vi "Initialize Plot.vi"(8 "error in (no error)":errorcluster, 10 "scale (1)":dbl=1.0, 11 "serial arm in":refnum<class "NI_Robotics_Serial Robot Arm.lvclass">) -> (0 "error out":errorcluster, 3 "serial arm out":refnum<class "NI_Robotics_Serial Robot Arm.lvclass">)   [LabVIEW 2017, in "NI_Robotics_3DKinematics.lvlib"]
doc: "Initializes a 3D object that represents a robotic arm."
uses:
  <vilib>/robotics/Kinematics/Plotting/NI_Robotics_3DKinematics.lvlib
  <vilib>/robotics/Kinematics/Robot/NI_Robotics_Serial Robot Arm.lvclass
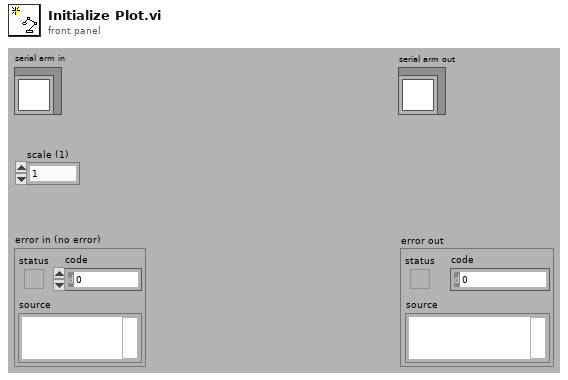
[diagram p1: front panel]
types:
  T1 = typedef "NI_Robotics_3DKinematics.lvlib/Tree Element.ctl" = cluster{"Name":string, "Parent":string, "Type":T2, "Visible?":bool, "Geometry Definition":dbl[], "Position WRT Parent (X,Y,Z)":dbl[], "Rotation WRT Parent (degrees)":dbl[], "Joint Type":T3, "Geometry File Path":path, "Indent Level":i32, "Color":u32}
  T2 = typedef "NI_Robotics_3DKinematics.lvlib/Element Type.ctl" = enum16{"Joint", "Box", "Cylinder", "Cone", "Sphere", "ASE File", "VRML File", "STL File", "Space"}
  T3 = typedef "NI_Robotics_3DKinematics.lvlib/Joint Type.ctl" = enum16{"Trans_X", "Trans_Y", "Trans_Z", "Rot_X", "Rot_Y", "Rot_Z", "None"}
  T4 = typedef "NI_Robotics_3DKinematics.lvlib/Joint Control.ctl" = cluster{"Joint Refnum":refnum<vi>, "Joint Type":T3, "Position WRT Parent":dbl[], "Rotation WRT Parent":dbl[], "Bar Refnum":refnum<vi>}
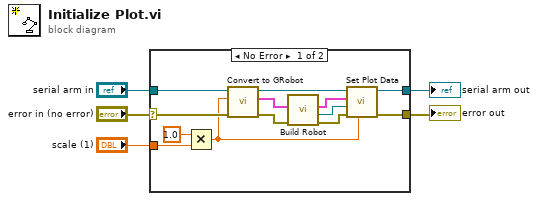
[diagram p0: block diagram]
diagram:
  n1 = case shown="No Error" "error in (no error)" {
    selector: "error in (no error)" -> [w13 w19]
    tunnel: "serial arm in" -> [w16 w20]
    tunnel: "scale (1)" -> [w14 _]
    tunnel: [w11 w19] -> w2
    tunnel: [w8 w20] -> w1
    frame No Error {
      n2 = Multiply(x=1.0, y=w14) -> (x*y=w6:dbl)
      n3 = call <vilib>:"Convert to GRobot.vi"("error in (no error)"=w13, "scale"=w6, "Robot In"=w16) -> ("error out"=w18:errorcluster, "Robot Elements"=w17:T1[], "Robot Out"=w10:refnum<class "NI_Robotics_Serial Robot Arm.lvclass">)  [unwired: 6 in]
      n4 = call <vilib>:"Build Robot.vi"("error in"=w18, "Robot Elements"=w17) -> ("error out"=w12:errorcluster, "Scene Out"=w7:refnum<vi>, "Joint Array"=w9:T4[])  [unwired: 7 in]
      n5 = call <vilib>:"Set Plot Data.vi"("Scale"=w6, "error in (no error)"=w12, "Serial Arm Scene"=w7, "Plot Data"=w9, "NI_Robotics_Serial Robot Arm in"=w10) -> ("error out"=w11:errorcluster, "NI_Robotics_Serial Robot Arm out"=w8:refnum<class "NI_Robotics_Serial Robot Arm.lvclass">)  [unwired: 5 in]
    }
    frame Error {
    }
  }
  "error out" <- w2
  "serial arm out" <- w1
